vi "S3859061_Task1.vi"() -> ()   [LabVIEW 2020]
panel:
  out "phi":dbl
  out "theta":dbl
  out "r":dbl
  in  "stop":bool
  in  "z":dbl
  in  "y":dbl
  in  "x":dbl
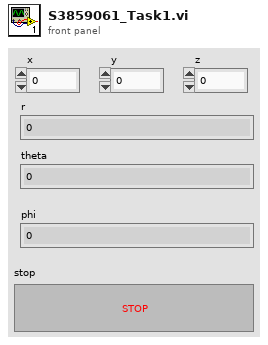
[diagram p1: front panel]
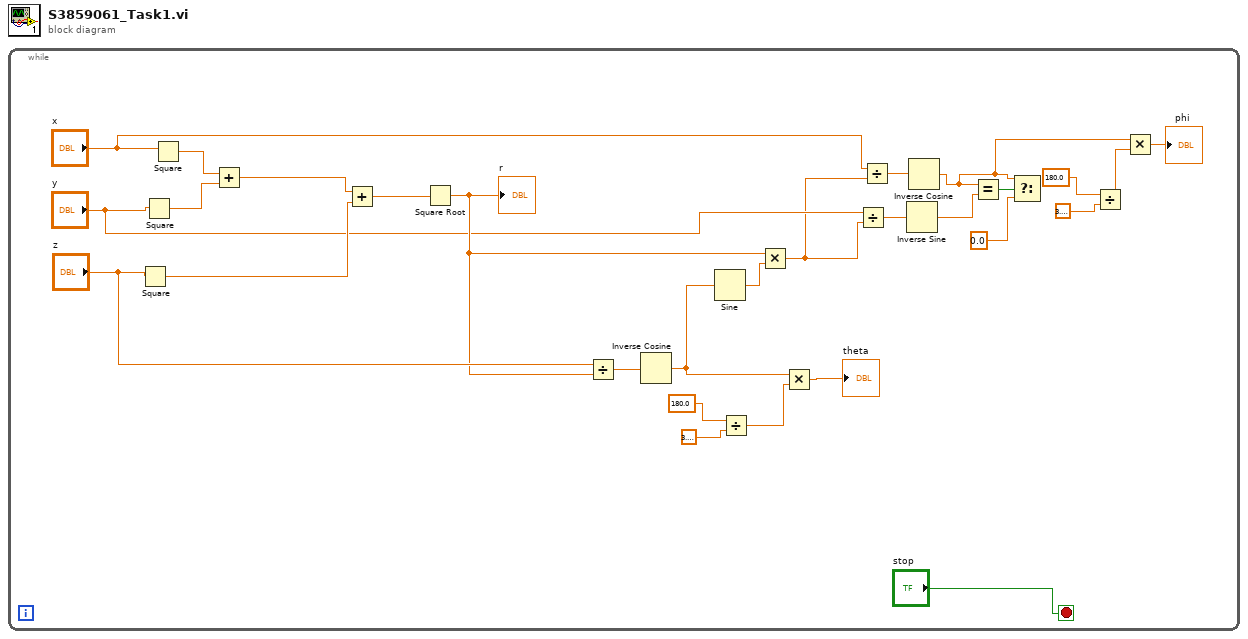
[diagram p0: block diagram]
diagram:
  n1 = while {
    stop <- "stop" stop-if-true
    n2 = Square(x="z") -> (x^2=w24:dbl)
    n3 = Square(x="y") -> (x^2=w26:dbl)
    n4 = Square(x="x") -> (x^2=w27:dbl)
    n5 = Add(x=w27, y=w26) -> (x+y=w25:dbl)
    n6 = Add(x=w25, y=w24) -> (x+y=w23:dbl)
    n7 = Square Root(x=w23) -> (sqrt(x)=w20:dbl)
    "r" <- w20
    n8 = Divide(x="z", y=w20) -> (x/y=w21:dbl)
    n9 = Inverse Cosine(1:w21) -> (0:w3:dbl)
    n10 = Sine(x=w3) -> (sin(x)=w19:dbl)
    n11 = Divide(x=180.0, y=3.141592653589793) -> (x/y=w2:dbl)
    n12 = Multiply(x=w20, y=w19) -> (x*y=w16:dbl)
    n13 = Multiply(x=w3, y=w2) -> (x*y=→"theta":dbl)
    n14 = Divide(x="y", y=w16) -> (x/y=w14:dbl)
    n15 = Divide(x="x", y=w16) -> (x/y=w15:dbl)
    n16 = Inverse Sine(1:w14) -> (0:w13:dbl)
    n17 = Inverse Cosine(1:w15) -> (0:w5:dbl)
    n18 = Equal?(x=w5, y=w13) -> (x = y?=w12:bool)
    n19 = Select(t=w5, s=w12, f=0.0) -> ()  [unwired: 1 out]
    n20 = Divide(x=180.0, y=3.141592653589793) -> (x/y=w6:dbl)
    n21 = Multiply(x=w5, y=w6) -> (x*y=→"phi":dbl)
  }
